vi "motor run.vi"(0 "PWM frequence":dbl=1250.0, 1 "PID gains":T1={"proportional gain (Kc)"=1.0, "integral time (Ti, min)"=0.01, "derivative time (Td, min)"=0.0} {"derivative time (Td, min)" format="%.3f"; "integral time (Ti, min)" format="%.3f"; "proportional gain (Kc)" format="%.3f"}, 4 "Motor.brake":bool, 5 "ratio":dbl, 7 "speed RPM":dbl, 9 "Reset":bool, 11 "error in":errorcluster, 12 "motor select":T2, 14 "dt(s)":dbl) -> (3 "setpoint":dbl, 6 "encoder":dbl, 10 "output":dbl format="%.2f", 15 "error out":errorcluster)   [LabVIEW 2019, in "my FPGA lib.lvlib" / "motor.lvlib"]
uses:
  motor.lvlib
  motor enum.ctl
  <vilib>/addons/control/pid/pid.llb/PID (DBL).vi
  my FPGA lib.lvlib
  <vilib>/addons/control/pid/NI_PID_pid.lvlib
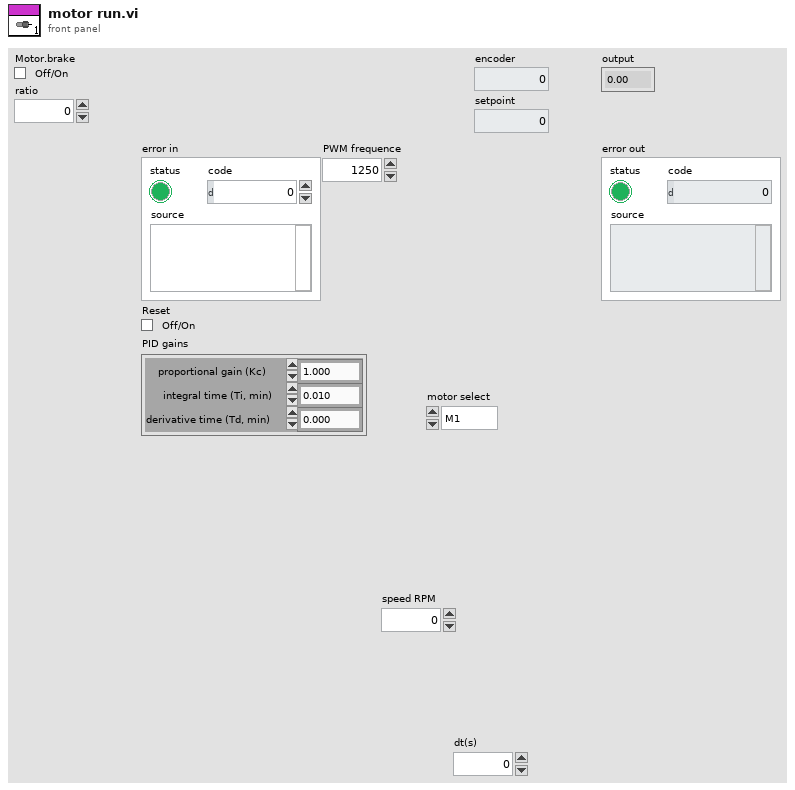
[diagram p1: front panel]
types:
  T1 = cluster{"proportional gain (Kc)":dbl, "integral time (Ti, min)":dbl, "derivative time (Td, min)":dbl}
  T2 = typedef "my FPGA lib.lvlib/motor.lvlib/motor enum.ctl" = enum16{"M1", "M2", "M3", "M4"}
  T3 = cluster{"divider rate":i32, "enable divider":bool, "period":i32}
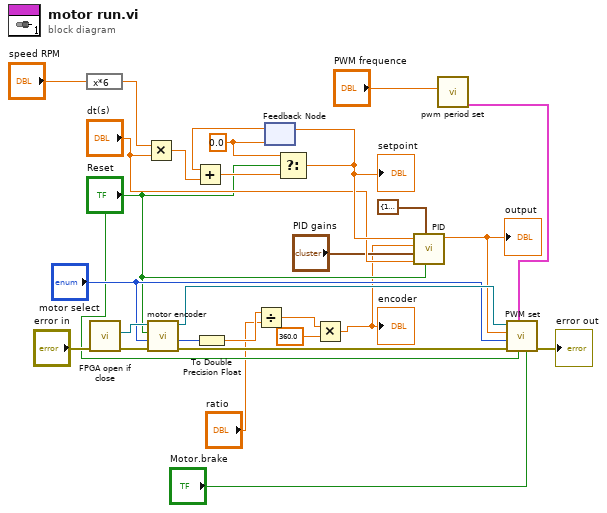
[diagram p0: block diagram]
diagram:
  w20 = 0.0 ("t")
  n1 = expression code="x*6"("speed RPM") -> (w23:dbl)
  n2 = call "FPGA open if close.vi"("error in"="error in") -> ("error out"=w27:errorcluster, "FPGA VI Reference Out"=w26:refnum<k20>)  [unwired: 9 in]
  n3 = Multiply(x=w23, y="dt(s)") -> (x*y=w19:dbl)
  n4 = call "motor encoder.vi"("Error In"=w27, "motor select"="motor select", "Reset"="Reset", "FPGA VI Reference In"=w26) -> ("error out"=w12:errorcluster, "encoder"=w25:i32, "FPGA VI Reference Out"=w13:refnum<k20>)  [unwired: 5 in]
  n5 = To Double Precision Float(number=w25) -> (double precision float=w2:dbl)
  n6 = Divide(x=w2, y="ratio") -> (x/y=w3:dbl)
  n7 = feedback #1(w20) -> (w21:dbl)
  n8 = Add(x=w21, y=w19) -> (x+y=w22:dbl)
  n9 = Select(t=w20, s="Reset", f=w22) -> (s? t:f=w18:dbl)
  "setpoint" <- w18
  n10 = feedback-in #1(w18) -> ()
  n11 = Multiply(x=w3, y=360.0) -> (x*y=w5:dbl)
  "encoder" <- w5
  n12 = call-poly <vilib>:"PID.vi"("reinitialize? (F)"="Reset", "output range"=cluster{"output high":dbl, "output low":dbl} {"output high"=100.0, "output low"=-100.0}, "dt (s)"="dt(s)", "PID gains"="PID gains", "process variable"=w5, "setpoint"=w18) -> ("output"=w11:dbl)  [unwired: 4 in, 1 out]
  "output" <- w11
  n13 = call "pwm period set.vi"("PWM frequence"="PWM frequence") -> ("pwm cnfg"=w9:T3)  [unwired: 10 in]
  n14 = call "PWM set.vi"("Motor.brake"="Motor.brake", "Reset"="Reset", "pwm cnfg"=w9, "Error In"=w12, "motor select"="motor select", "PWM"=w11, "FPGA VI Reference In"=w13) -> ("error out"=→"error out":errorcluster)  [unwired: 4 in]
